vi "5-2.vi"() -> ()   [LabVIEW 2019, in "5.lvlib"]
uses:
  5.lvlib
panel:
  out "sum":i16
  out "Array":i32[][](array[numeric])
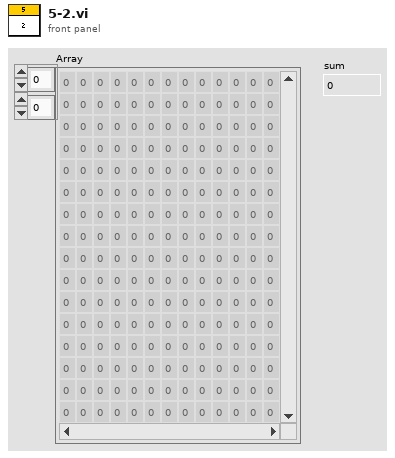
[diagram p1: front panel]
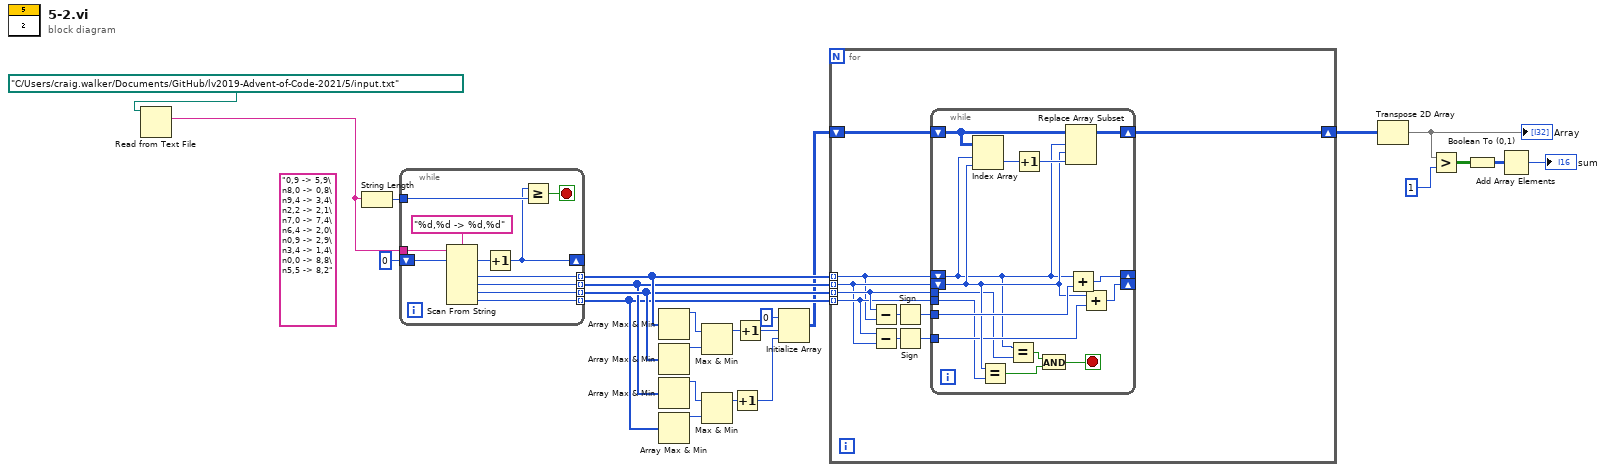
[diagram p0: block diagram]
diagram:
  (unwired) "0,9 -> 5,9\n8,0 -> 0,8\n9,4 -> 3,4\n2,2 -> 2,1\n7,0 -> 7,4\n6,4 -> 2,0\n0,9 -> 2,9\n3,4 -> 1,4\n0,0 -> 8,8\n5,5 -> 8,2"
  n1 = Read from Text File(file (use dialog)=path "C:/Users/craig.walker/Documents/GitHub/lv2019-Advent-of-Code-2021/5/input.txt" ("file path (dialog if empty)")) -> (text=w1:string)  [unwired: 3 in, 3 out]
  n2 = String Length(string=w1) -> (length=w23:i32)
  n3 = while {
    tunnel: w1 -> [w35]
    shift-right: [w25] -> _
    shift-left: u32 0 -> [w34]
    tunnel: w23 -> [w27]
    tunnel: [w31] -> w20 mode=indexing
    tunnel: [w30] -> w12 mode=indexing
    tunnel: [w29] -> w19 mode=indexing
    tunnel: [w28] -> w11 mode=indexing
    stop <- w33 stop-if-true
    n4 = Scan From String(format string="%d,%d -> %d,%d", input string=w35, initial scan location=w34) -> (offset past scan=w26:u32, output 1=w31:i32, output 2=w30:i32, output 3=w29:i32, output 4=w28:i32)  [unwired: 5 in, 2 out]
    n5 = Increment(x=w26) -> (x+1=w25:u32)
    n6 = Greater Or Equal?(x=w25, y=w27) -> (x >= y?=w33:bool)
  }
  n7 = Array Max & Min(array=w20) -> (max value=w18:i32)  [unwired: 3 out]
  n8 = Array Max & Min(array=w19) -> (max value=w17:i32)  [unwired: 3 out]
  n9 = Array Max & Min(array=w12) -> (max value=w13:i32)  [unwired: 3 out]
  n10 = Array Max & Min(array=w11) -> (max value=w14:i32)  [unwired: 3 out]
  n11 = Max & Min(x=w18, y=w17) -> (max(x,y)=w15:i32)  [unwired: 1 out]
  n12 = Max & Min(x=w13, y=w14) -> (max(x,y)=w10:i32)  [unwired: 1 out]
  n13 = Increment(x=w10) -> (x+1=w7:i32)
  n14 = Increment(x=w15) -> (x+1=w8:i32)
  n15 = Initialize Array(0, w8, w7) -> (w9:i32[][])
  n16 = for {
    shift-right: [w44] -> w21
    shift-left: w9 -> [w45]
    tunnel: w20 -> [w40] mode=indexing
    tunnel: w12 -> [w41] mode=indexing
    tunnel: w19 -> [w43] mode=indexing
    tunnel: w11 -> [w42] mode=indexing
    n17 = Subtract(x=w43, y=w40) -> (x-y=w39:i32)
    n18 = Subtract(x=w42, y=w41) -> (x-y=w37:i32)
    n19 = Sign(1:w39) -> (0:w38:i32)
    n20 = Sign(1:w37) -> (0:w36:i32)
    n21 = while {
      shift-right: [w60] -> w44
      shift-left: w45 -> [w59]
      tunnel: w43 -> [w47]
      tunnel: w42 -> [w46]
      shift-right: [w56] -> _
      shift-left: w40 -> [w51]
      shift-right: [w55] -> _
      shift-left: w41 -> [w53]
      tunnel: w38 -> [w54]
      tunnel: w36 -> [w52]
      stop <- w48 stop-if-true
      n22 = Index Array(array=w59, index (row)=w51, index (col)=w53) -> (element=w58:i32)
      n23 = Equal?(x=w53, y=w46) -> (x = y?=w49:bool)
      n24 = Equal?(x=w51, y=w47) -> (x = y?=w50:bool)
      n25 = Increment(x=w58) -> (x+1=w57:i32)
      n26 = And(x=w50, y=w49) -> (x .and. y?=w48:bool)
      n27 = Replace Array Subset(array=w59, new element=w57, index (row)=w51, index (col)=w53) -> (w60:i32[][])
      n28 = Add(x=w51, y=w54) -> (x+y=w56:i32)
      n29 = Add(x=w53, y=w52) -> (x+y=w55:i32)
    }
  }
  n30 = Transpose 2D Array(2D array=w21) -> (transposed array=w6:i32[][])
  "Array" <- w6
  n31 = Greater?(x=w6, y=1) -> (0:w4:bool[][])
  n32 = Boolean To (0,1)(Boolean=w4) -> (0, 1=w3:i16[][])
  n33 = Add Array Elements(numeric array=w3) -> (sum=→"sum":i16)
